vi "Drive Controller.vi"(8 "error in":errorcluster) -> ()   [LabVIEW 2017]
doc: "This VI executes continuously carrying out the current operation and responding to updates or new operation requests. It will often contain the timing or control code that is difficult to place directly in TeleOp. This VI generally opens all sensors and motors and isolates the rest of the robot code from knowing implementation details of how the operations are carried out."
uses:
  <vilib>/Rock Robotics/WPI/Framework/Completion Status.ctl
  Drive Setpoints.ctl
  Drive Operations.ctl
  <vilib>/Rock Robotics/WPI/SafetyOutput/WPI_SafetyOutputConfigMenu.ctl
  <vilib>/Rock Robotics/SystemInterfaces/DIO/FPGA_DIOPWMChannel.ctl
  <vilib>/Rock Robotics/WPI/RobotDrive/WPI_RobotDriveOpen4MotorWithTalonSRX.vi
panel:
  in  "Interactive Values":T1
  in  "Buttons":cluster{"Execute Cmd":bool, "Abort Cmd":bool}
  out "Command Timing":cluster{"Start Time (ms)":u32, "Iterations":i32}
  out "Status":T3
  out "Setpoints":T4(graph)
  out "Current\nCmd":string
  # "Tip: The graph shows the motor setpoints. It may also be helpful to observe inputs and sensor values.\nYou may also want to display tuning or debugging controls."
  # "Interactive Command: You may fill in the settings for a command\nand schedule it with the Execute button. You can observe and abort\nany command while fine tuning the code for the controller."
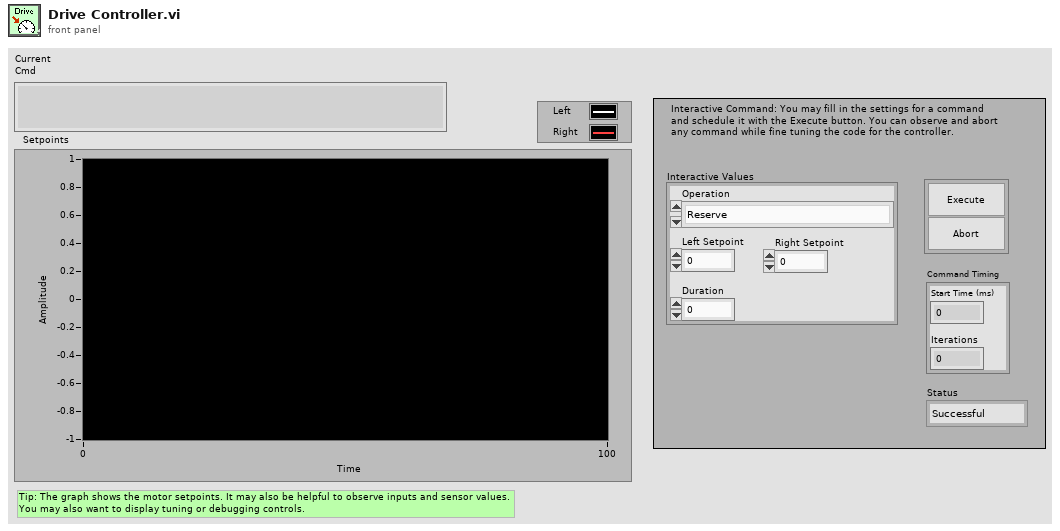
[diagram p1: front panel]
types:
  T1 = typedef "Drive Setpoints.ctl" = cluster{"Operation":T2, "Left Setpoint":dbl, "Right Setpoint":dbl, "Duration":dbl}
  T2 = typedef "Drive Operations.ctl" = enum16{"Reserve", "Read Current", "Immediate", "Drive for Time", "Drive for Distance"}
  T3 = typedef "Completion Status.ctl" = enum16{"Successful", "Aborted", "Incomplete"}
  T4 = cluster{"Left Setpoint":dbl, "Right Setpoint":dbl}
  T5 = typedef "FPGA_DIOPWMChannel.ctl" = enum8{"PWM 0", "PWM 1", "PWM 2", "PWM 3", "PWM 4", "PWM 5", "PWM 6", "PWM 7", "PWM 8", "PWM 9", "PWM MXP 0", "PWM MXP 1", "PWM MXP 2", "PWM MXP 3", "PWM MXP 4", "PWM MXP 5", "PWM MXP 6", "PWM MXP 7", "PWM MXP 8", "PWM MXP 9", "Invalid"}
  T6 = typedef "WPI_SafetyOutputConfigMenu.ctl" = enum16{"Enable", "Disable"}
  T7 = typedef "WPI_RobotDriveDevRef.ctl" = cluster{"DevStatus":errorcluster, "Motors[]":T8[], "Square Inputs":bool, "Max Output":dbl}
  T8 = typedef "WPI_MotorControlDeviceRef.ctl" = cluster{"DeviceStatus":errorcluster, "Type":T9, "PWM":cluster{"PWM Channel":T5, "DeadBand":T10}, "CAN":cluster{"Device Number":u8, "SetOutput VI Ref":variant, "GetOutput VI Ref":variant, "Enable VI Ref":variant, "Disable VI Ref":variant, "Data":variant}, "Invert":bool, "DIO PWM":cluster{"PWM \"Enable\" Channel":T5, "DIOChannel":T11, "PWM Rate":dbl}}
  T9 = typedef "WPI_MotorControlType.ctl" = enum16{"PWM", "CAN", "DIO PWM"}
  T10 = typedef "WPI_PWMDeadband.ctl" = cluster{"Name":string, "maxPositivePwm":i32, "minPositivePwm":i32, "centerPwm":i32, "maxNegativePwm":i32, "minNegativePwm":i32, "angularRange":u16}
  T11 = typedef "FPGA_DIOChannel.ctl" = enum8{"DIO 0", "DIO 1", "DIO 2", "DIO 3", "DIO 4", "DIO 5", "DIO 6", "DIO 7", "DIO 8", "DIO 9", "DIO MXP 0", "DIO MXP 1", "DIO MXP 2", "DIO MXP 3", "DIO MXP 4", "DIO MXP 5", "DIO MXP 6", "DIO MXP 7", "DIO MXP 8", "DIO MXP 9", "DIO MXP 10", "DIO MXP 11", "DIO MXP 12", "DIO MXP 13", "DIO MXP 14", "DIO MXP 15", "SPI Port CS1", "SPI Port CS2", "SPI Port CS3", "SPI Port MISO", "SPI Port MOSI", "Invalid"}
  T12 = typedef "Command Status Info.ctl" = cluster{"Name":string, "Status":T3, "notifier out":T13}
  T13 = typedef "Completion Notifier.ctl" = refnum<notifier>
  T14 = cluster{"SubSystem Data":T1, cluster{"Start Time (ms)":u32, "Iterations":i32}, cluster{"Command Info":T12, "Description":string, "Default Command":T1, "queue out":refnum<queue>, "Subsystem Name":string}}
  T15 = cluster{"SubSystem Data":T1, cluster{"Start Time (ms)":u32, "Iterations":i32}, "Default Command Arguments":cluster{"Command Info":T12, "Description":string, "Default Command":T1, "queue out":refnum<queue>, "Subsystem Name":string}}
  T16 = cluster{"Don't move motors while reserved":dbl, "Don't move motors while reserved":dbl}
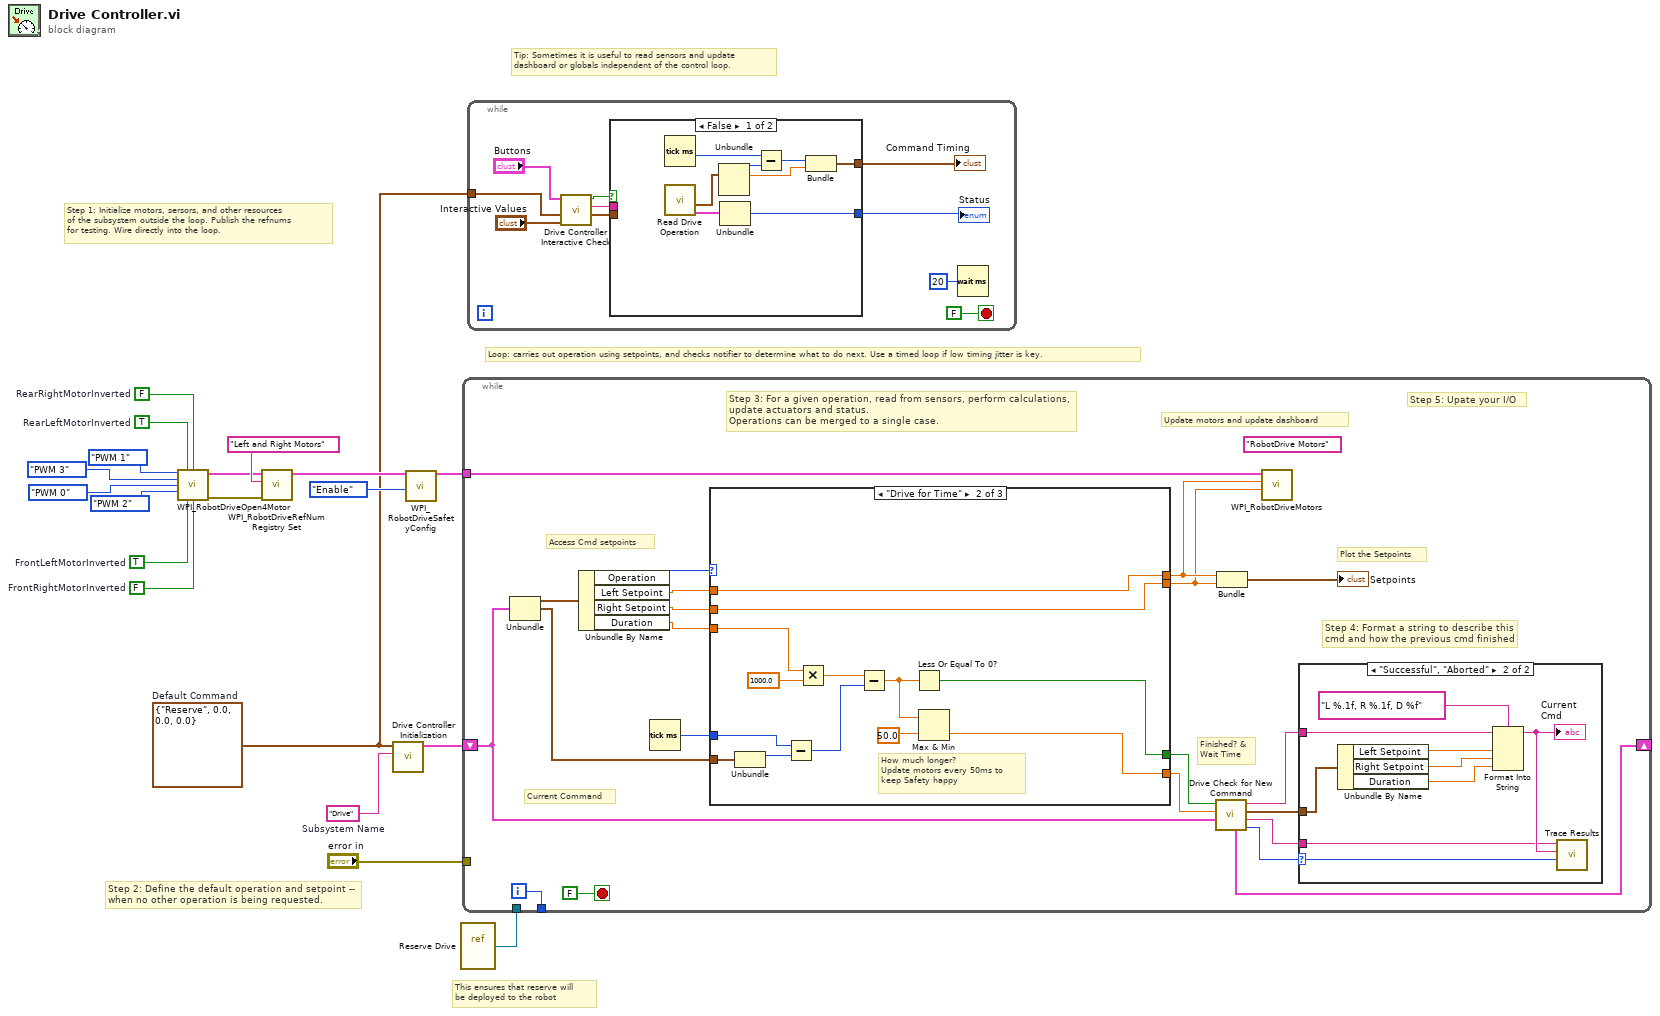
[diagram p0: block diagram]
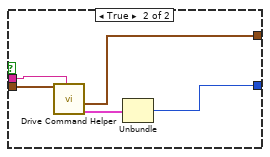
[diagram p2: hidden frame]
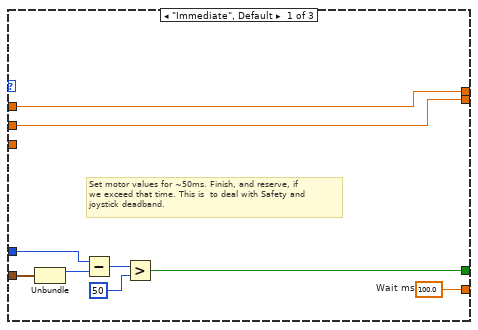
[diagram p4: hidden frame]
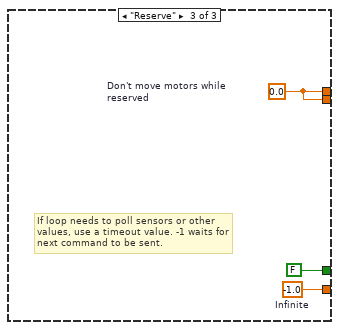
[diagram p5: hidden frame]
diagram:
  w10 = TRUE  # FrontLeftMotorInverted
  w7 = FALSE  # FrontRightMotorInverted
  w9 = TRUE  # RearLeftMotorInverted
  w8 = FALSE  # RearRightMotorInverted
  w11 = T1 {"Operation"=enum."Reserve", "Left Setpoint"=0.0, "Right Setpoint"=0.0, "Duration"=0.0}  # Default Command
  w19 = "Drive"  # Subsystem Name
  # "This ensures that reserve will\nbe deployed to the robot"
  # "Tip: Sometimes it is useful to read sensors and update\ndashboard or globals independent of the control loop."
  # "Step 2: Define the default operation and setpoint --\nwhen no other operation is being requested."
  # "Step 1: Initialize motors, sersors, and other resources\nof the subsystem outside the loop. Publish the refnums\nfor testing. Wire directly into the loop."
  # "Loop: carries out operation using setpoints, and checks notifier to determine what to do next. Use a timed loop if low timing jitter is key."
  n1 = call-poly <vilib>:"WPI_RobotDriveOpen4Motor.vi"("Rear Left Motor"=FPGA_DIOPWMChannel."PWM 1" ("Rear Right Motor"), "Rear Left Motor Inverted"=w9, "Rear Right Motor Inverted"=w8, "Rear Right Motor"=FPGA_DIOPWMChannel."PWM 3" ("Front Left Motor"), "Front Left Motor"=FPGA_DIOPWMChannel."PWM 0" ("Rear Left Motor"), "Front Right Motor"=FPGA_DIOPWMChannel."PWM 2", "Front Left Motor Inverted"=w10, "Front Right Motor Inverted"=w7) -> ("RobotDriveDevRef"=w6:T7, "error out"=w5:errorcluster)  [unwired: 6 in]
  n2 = call <vilib>:"WPI_RobotDriveRefNum Registry Set.vi"("error in (no error)"=w5, "refnum name"="Left and Right Motors", "RobotDriveDevRef"=w6) -> ("RobotDriveDevRef"=w17:T7)  [unwired: 1 in, 7 out]
  n3 = call "Drive Controller Initialization.vi"("Subsystem Name"=w19, "Default Command"=w11) -> ("Current Command"=w13:T14)  [unwired: 9 in]
  n4 = call <vilib>:"WPI_RobotDriveSafetyConfig.vi"("mode"=WPI_SafetyOutputConfigMenu."Enable", "RobotDriveDevRef"=w17) -> ("RobotDriveDevRef"=w15:T7)  [unwired: 8 in, 1 out]
  n5 = vi-ref "Reserve Drive.vi"() -> (w12:refnum<vi>)
  n6 = while {
    shift-right: [w27] -> _
    shift-left: w13 -> [w20]
    tunnel: [w39] -> _
    tunnel: w15 -> [w35]
    tunnel: "error in" -> [_]
    tunnel: w12 -> [_]
    i -> [w39]
    stop <- FALSE stop-if-true
    (unwired) "RobotDrive Motors" ("Name")
    # "Step 5: Upate your I/O"
    # "Step 4: Format a string to describe this\ncmd and how the previous cmd finished"
    # "Current Command"
    # "Update motors and update dashboard"
    # "Plot the Setpoints"
    # "Access Cmd setpoints"
    # "Finished? &\nWait Time"
    # "Step 3: For a given operation, read from sensors, perform calculations,\nupdate actuators and status.\nOperations can be merged to a single case."
    n7 = Unbundle(w20) -> ("SubSystem Data"=w34:T1, w21:cluster{"Start Time (ms)":u32, "Iterations":i32})  [unwired: 1 out]
    n8 = Unbundle By Name(w34) -> ("Operation"=w33:T2, "Left Setpoint"=w32:dbl, "Right Setpoint"=w31:dbl, "Duration"=w30:dbl)
    n9 = Tick Count (ms)() -> (millisecond timer value=w29:u32)
    n10 = case shown="\"Drive for Time\"" w33 {
      tunnel: [w58 w59 w74] -> w26
      tunnel: [w51 w66 FALSE ("ignore previous (F)")] -> w25
      tunnel: w21 -> [w50 w68 _]
      tunnel: [w57 w65 w72] -> w37
      tunnel: [w56 w64 w72] -> w36
      tunnel: w32 -> [w57 w65 _]
      tunnel: w31 -> [w56 w64 _]
      tunnel: w30 -> [_ w63 _]
      tunnel: w29 -> [w52 w62 _]
      frame "Immediate", Default {
        w58 = 100.0  # Wait ms
        # "Set motor values for ~50ms. Finish, and reserve, if\nwe exceed that time. This is  to deal with Safety and\njoystick deadband."
        n11 = Unbundle(w50) -> ("Start Time (ms)"=w53:u32)  [unwired: 1 out]
        n12 = Subtract(x=w52, y=w53) -> (x-y=w54:u32)
        n13 = Greater?(x=w54, y=u8 50 ("Left Motor")) -> (0:w51:bool)
      }
      frame "Drive for Time" {
        # "How much longer?\nUpdate motors every 50ms to\nkeep Safety happy"
        n14 = Unbundle(w68) -> ("Start Time (ms)"=w67:u32)  [unwired: 1 out]
        n15 = Subtract(x=w62, y=w67) -> (x-y=w71:u32)
        n16 = Multiply(x=w63, y=1000.0) -> (x*y=w70:dbl)
        n17 = Subtract(x=w70, y=w71) -> (x-y=w61:dbl)
        n18 = Less Or Equal To 0?(x=w61) -> (x <= 0?=w66:bool)
        n19 = Max & Min(x=w61, y=50.0) -> (min(x,y)=w59:dbl)  [unwired: 1 out]
      }
      frame "Reserve" {
        w72 = 0.0  # Don't move motors while reserved
        w74 = -1.0  # Infinite
        # "If loop needs to poll sensors or other\nvalues, use a timeout value. -1 waits for\nnext command to be sent."
      }
    }
    n20 = call "Drive Check for New Command.vi"("input cluster"=w20, "Wait time (ms)"=w26, "Finished?"=w25) -> ("Completion"=w28:T3, "Subsystem Name"=w22:string, "Current Command"=w23:T1, "Initial Trace String"=w24:string, "Next Command"=w27:T15)  [unwired: 4 in]
    n21 = Bundle("Don't move motors while reserved"=w37, "Don't move motors while reserved"=w36) -> (→"Setpoints":T16)  [unwired: 1 in]
    n22 = call <vilib>:"WPI_RobotDriveMotors.vi"("RightSpeed"=w36, "LeftSpeed"=w37, "RobotDriveDevRef"=w35) -> ()  [unwired: 1 in, 8 out]
    n23 = case shown="\"Successful\", \"Aborted\"" w28 {
      selector: w28 -> [_ w49]
      tunnel: w24 -> [_ w44]
      tunnel: w23 -> [_ w45]
      tunnel: w22 -> [_ w41]
      frame "Incomplete", Default {
        # "Continuing current command"
      }
      frame "Successful", "Aborted" {
        # "Report and setup for next command"
        n24 = Unbundle By Name(w45) -> ("Left Setpoint"=w47:dbl, "Right Setpoint"=w48:dbl, "Duration"=w42:dbl)
        n25 = Format Into String(format string="L %.1f, R %.1f, D %f", initial string=w44, w47, w48, w42) -> (resulting string=w43:string)  [unwired: 1 in, 1 out]
        "Current\nCmd" <- w43
        n26 = call <vilib>:"Trace Results.vi"("Status of previous command"=w49, "Description"=w43, "Subsystem"=w41) -> ()  [unwired: 9 in]
      }
    }
  }
  n27 = while {
    tunnel: w11 -> [w76]
    stop <- FALSE stop-if-true
    n28 = call "Drive Controller Interactive Check.vi"("Interactive Command In"="Interactive Values", "Default Command"=w76, "Buttons"="Buttons") -> ("Interactive Command Out"=w78:T1, "Trace String"=w79:string, "Schedule"=w80:bool)  [unwired: 6 in]
    n29 = case shown="False" w80 {
      tunnel: [w89 w97] -> w81
      tunnel: [w88 w93] -> w82
      tunnel: w79 -> [_ w95]
      tunnel: w78 -> [_ w94]
      frame False {
        n30 = Tick Count (ms)() -> (millisecond timer value=w92:u32)
        n31 = call "Read Drive Operation.vi"() -> ("Command Info"=w86:T12, "SubSystem Data"=w85:T1)  [unwired: 9 in, 1 out]
        n32 = Unbundle(w85) -> ("Operation"=w90:T2, "Left Setpoint"=w87:dbl)  [unwired: 2 out]
        n33 = Unbundle(w86) -> ("Status"=w89:T3)  [unwired: 2 out]
        n34 = Subtract(x=w92, y=w90) -> (x-y=w91:u32)
        n35 = Bundle(w91, "Left Setpoint"=w87) -> (w88:cluster{u32, "Left Setpoint":dbl})  [unwired: 1 in]
      }
      frame True {
        n36 = call "Drive Command Helper.vi"("Description"=w95, "SubSystem Data"=w94) -> ("Command Info Out"=w96:T12, "Command Timing"=w93:cluster{"Start Time (ms)":u32, "Iterations":i32})  [unwired: 7 in, 1 out]
        n37 = Unbundle(w96) -> ("Status"=w97:T3)  [unwired: 2 out]
      }
    }
    "Status" <- w81
    "Command Timing" <- w82
    n38 = Wait (ms)(milliseconds to wait=u32 20) -> ()  [unwired: 1 out]
  }
